vi "Create Connection Handler.vi"(5 "ConnectionHandler in":refnum<class "ConnectionHandler.lvclass">, 8 "error in (no error)":errorcluster, 10 "Connection Configuration":refnum<class "Connection.lvclass">, 11 "Request":refnum<queue>) -> (0 "error out":errorcluster, 3 "ConnectionHandler":refnum<class "ConnectionHandler.lvclass">)   [LabVIEW 2013, in "MQTT_Connection.lvlib" / "ConnectionHandler.lvclass"]
uses:
  ConnectionHandler.lvclass
  MQTT_Base/Base Class/Request -- cluster.ctl
  <vilib>/LabVIEW Open Source Project/MQTT Control Packets/Control Packets/ControlPacket/ControlPacket.lvclass
  MQTT_Base/Base Class/Response -- cluster.ctl
  Connection/Connection.lvclass
  ConnectionHandler.lvclass/ConnectionHandler.ctl
  MQTT_Base/Base Class/MQTT_Base.lvclass
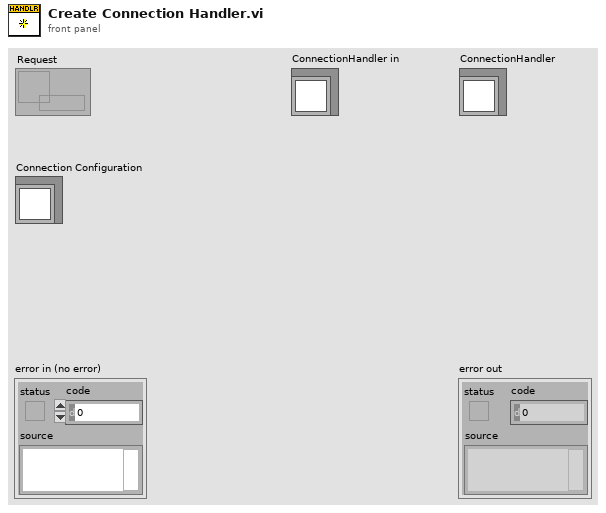
[diagram p1: front panel]
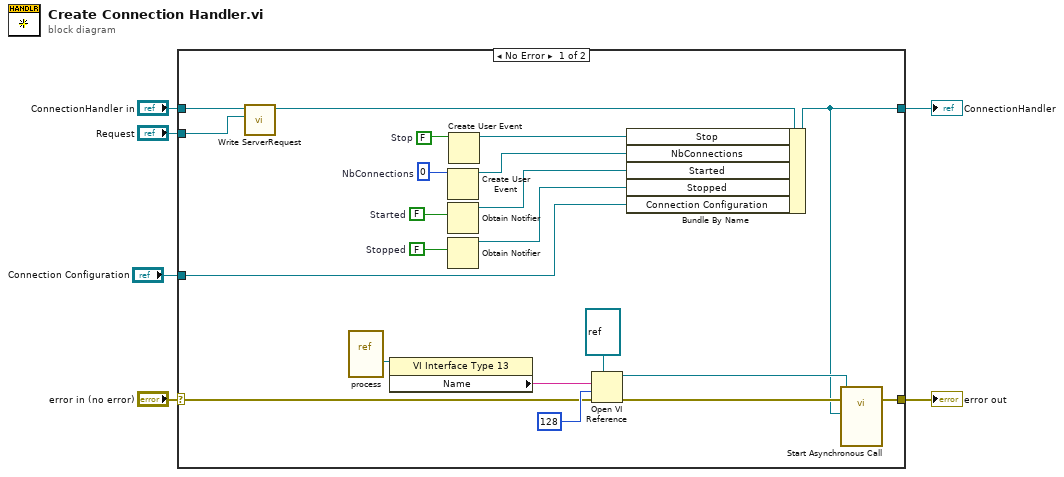
[diagram p0: block diagram]
diagram:
  n1 = case shown="No Error" "error in (no error)" {
    selector: "error in (no error)" -> [w14 w29]
    tunnel: [w13 w29] -> w5
    tunnel: [w17 w28] -> w3
    tunnel: "ConnectionHandler in" -> [w26 w28]
    tunnel: "Request" -> [w27 _]
    tunnel: "Connection Configuration" -> [w8 _]
    frame No Error {
      w12 = u32 0  # NbConnections
      w15 = FALSE  # Stopped
      w16 = FALSE  # Started
      w25 = FALSE  # Stop
      n2 = call "Write ServerRequest.vi"("ServerRequest"=w27, "TCPConnectionHandler in"=w26) -> ("TCPConnectionHandler out"=w23:refnum<class "ConnectionHandler.lvclass">)  [unwired: 9 in]
      n3 = vi-ref "process.vi"() -> (w22:refnum<vi>)
      n4 = property class="VI Interface Type 13"(reference=w22) -> ("Name"=w21:string)  [unwired: 1 in, 2 out]
      n5 = Create User Event(user event datatype=w12) -> (user event=w11:refnum<user-event>)  [unwired: 1 in, 1 out]
      n6 = Obtain Notifier(notification data type=w16) -> (notifier out=w10:refnum<notifier>)  [unwired: 3 in, 2 out]
      n7 = Obtain Notifier(notification data type=w15) -> (notifier out=w9:refnum<notifier>)  [unwired: 3 in, 2 out]
      n8 = Create User Event(user event datatype=w25) -> (user event=w24:refnum<user-event>)  [unwired: 1 in, 1 out]
      n9 = Open VI Reference(type specifier VI Refnum (for type only)=refnum<vi> refnum ("reference out"), vi path=w21, options=128, error in (no error)=w14) -> (vi reference=w20:refnum<vi>, error out=w19:errorcluster)  [unwired: 2 in]
      n10 = Bundle By Name(cluster=w23, "Stop"=w24, "NbConnections"=w11, "Started"=w10, "Stopped"=w9, "Connection Configuration"=w8) -> (w17:refnum<class "ConnectionHandler.lvclass">)
      n11 = call-by-ref "Start Asynchronous Call"(reference=w20, error in=w19, "ConnectionHandler in"=w17) -> (error out=w13:errorcluster)  [unwired: 9 in, 3 out]
    }
    frame Error {
    }
  }
  "error out" <- w5
  "ConnectionHandler" <- w3
